vi "Main.vi"(11 "Module Admin":refnum<class "Delacor_lib_QMH_Module Admin.lvclass">) -> ()   [LabVIEW 2020, in "Logging.lvlib"]
doc: "This template is based off of the Queued Message Handler design pattern and the Queued Message Handler project template that ships with LabVIEW.\n\nThe main difference is that the queue is private to this module and communication between modules is performed via Broadcast and Request events.\n\nRequest events are wrapped in public API methods and are handled in the Event Handling Loop (EHL) of this VI. Any module can register for Broadcast events sent by this module. The EHL generates messages based on user interface actions.\n\nThe Message Handling Loop (MHL) processes messages generated by the EHL, or by other messages. The messages are string values, so new messages can be added easily to the Message Cases case structure in the MHL. Each message cluster can also provide an optional value for Message Data, which is a variant that can be converted to whatever message-specific data is required.\n_____\nBased on Delacor QMH Project Template 6.0.0.89."
uses:
  Logging.lvlib
  <vilib>/Delacor/Delacor QMH/Libraries/Module Admin_class/Delacor_lib_QMH_Module Admin.lvclass
  Module Data--cluster.ctl
  Stop Argument--cluster.ctl
  <vilib>/Delacor/Delacor QMH/Libraries/Message Queue_class/Delacor_lib_QMH_Message Queue.lvclass/Delacor_lib_QMH_Message Queue.ctl
  <vilib>/Delacor/Delacor QMH/Libraries/Module Admin_class/Delacor_lib_QMH_Module Admin.lvclass/Delacor_lib_QMH_Module Admin.ctl
  save tdms Argument--cluster.ctl
  <vilib>/Utility/miscctls.llb/LVPointTypeDef.ctl
  <vilib>/Delacor/Delacor QMH/Libraries/Message Queue_class/Delacor_lib_QMH_Enqueue Message (Single).vi
  <vilib>/Delacor/Delacor QMH/Libraries/Module Admin_class/Delacor_lib_QMH_Get External Launch.vi
  <vilib>/Utility/error.llb/Error Cluster From Error Code.vi
  <vilib>/ErrorRing/Error Ring.xnode
  <vilib>/Delacor/Delacor QMH/Libraries/Message Queue_class/Delacor_lib_QMH_Message Queue.lvclass
  Settings/Settings.lvlib
  Acquisition/Acquisition .lvlib
panel:
  out "data":waveform(dbl)[](array[waveform])
  in  "Save Button":bool
  out "error out":errorcluster
  out "Status":string
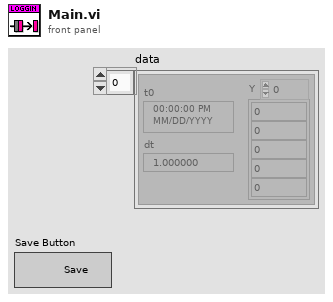
[diagram p1: front panel]
types:
  T1 = typedef "Logging.lvlib/Request Events--cluster.ctl" = cluster{"Stop Module":refnum<user-event>, "Show Panel":refnum<user-event>, "Hide Panel":refnum<user-event>, "Get Module Execution Status":refnum<user-event>, "Show Diagram":refnum<user-event>, "save tdms":refnum<user-event>}
  T2 = typedef "Acquisition .lvlib/Broadcast Events--cluster.ctl" = cluster{"Module Did Init":refnum<user-event>, "Status Updated":refnum<user-event>, "Error Reported":refnum<user-event>, "Module Did Stop":refnum<user-event>, "Update Module Execution Status":refnum<user-event>, "analog data":refnum<user-event>, "digital data":refnum<user-event>, "Digital Metdata has been acquired":refnum<user-event>}
  T3 = typedef "Settings.lvlib/Broadcast Events--cluster.ctl" = cluster{"Module Did Init":refnum<user-event>, "Status Updated":refnum<user-event>, "Error Reported":refnum<user-event>, "Module Did Stop":refnum<user-event>, "Update Module Execution Status":refnum<user-event>, "Config has been set":refnum<user-event>, "Prueba has been set":refnum<user-event>, "Digital has been set":refnum<user-event>}
  T4 = typedef "Logging.lvlib/Module Data--cluster.ctl" = cluster{"Status":string, "Nombre de la Prueba":string, "data":waveform(dbl)[], "data 2":u8[]}
  T5 = enum32{"invalid lock state", "Not Locked", "Locked (No Password)", "Password-protected"}
  T6 = typedef "Logging.lvlib/Stop Argument--cluster.ctl" = cluster{"Origin":string, "Exit via Stop Module Req?":bool, "Wait for Module to stop?":bool}
  T7 = typedef "Logging.lvlib/save tdms Argument--cluster.ctl" = cluster{"Boolean":bool}
  T8 = typedef "LVPointTypeDef.ctl" = cluster{"Horizontal":i16, "Vertical":i16}
  T9 = enum32{"Invalid", "Standard", "Closed", "Hidden", "Minimized", "Maximized"}
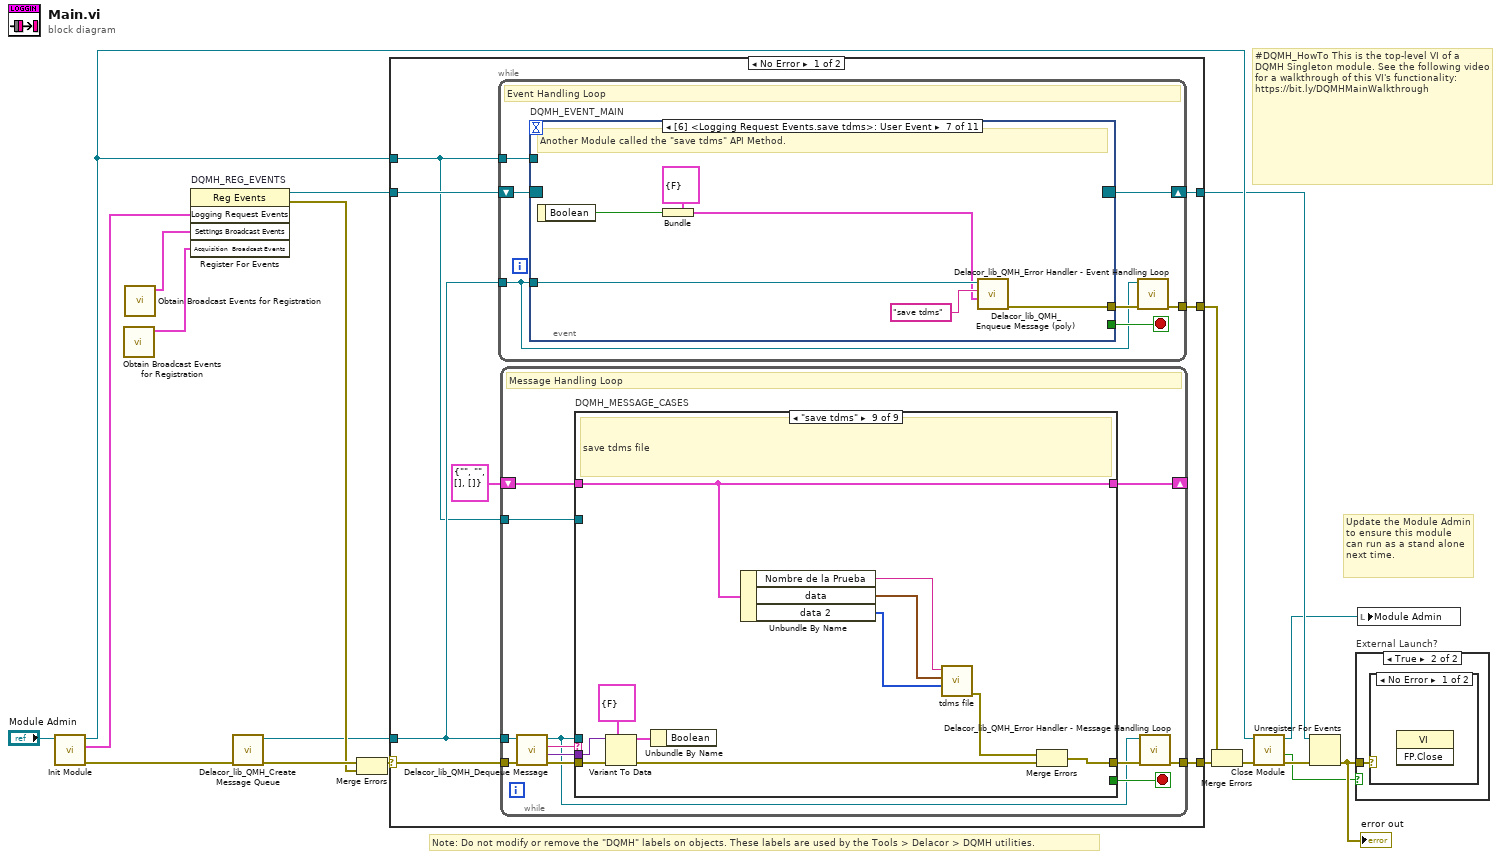
[diagram p0: block diagram]
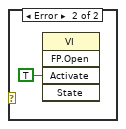
[diagram p3: hidden frame]
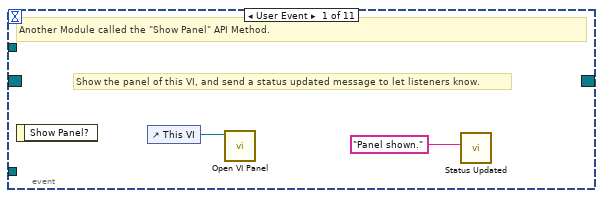
[diagram p4: hidden frame]
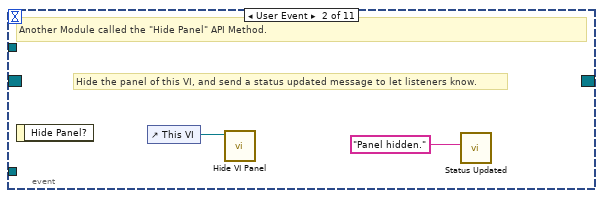
[diagram p5: hidden frame]
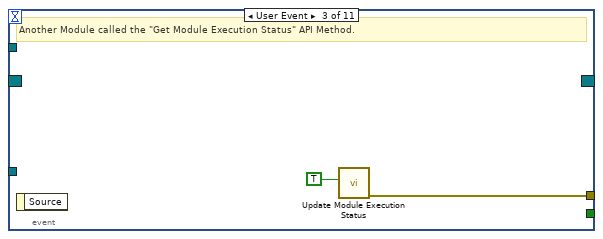
[diagram p6: hidden frame]
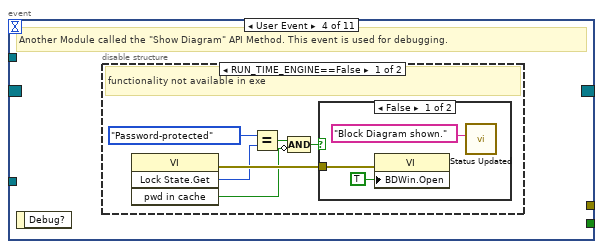
[diagram p7: hidden frame]
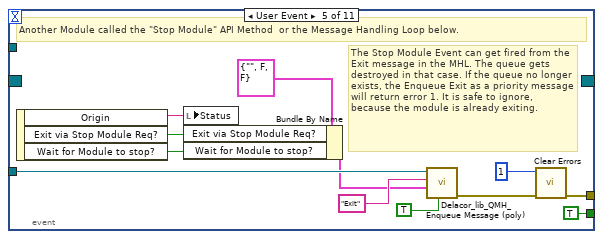
[diagram p10: hidden frame]
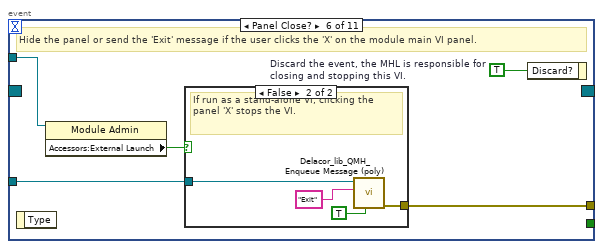
[diagram p11: hidden frame]
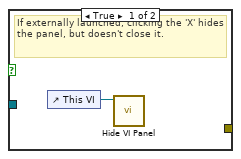
[diagram p12: hidden frame]
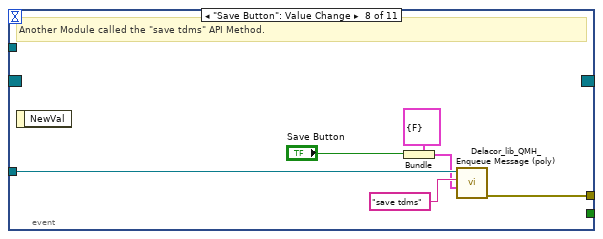
[diagram p13: hidden frame]
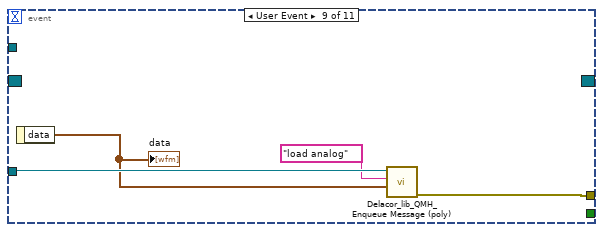
[diagram p14: hidden frame]
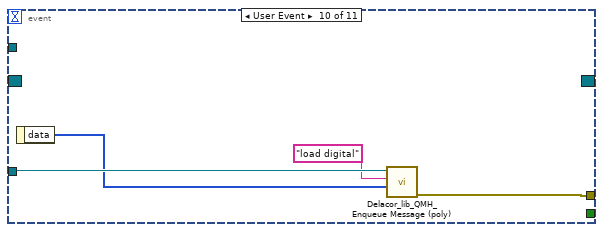
[diagram p15: hidden frame]
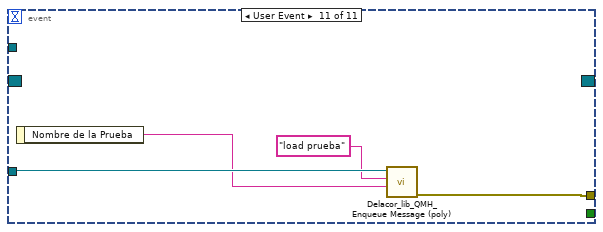
[diagram p16: hidden frame]
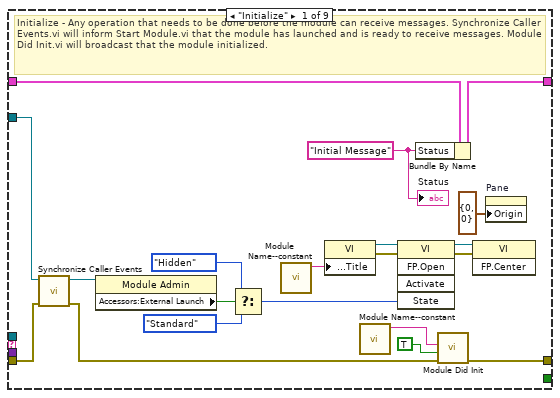
[diagram p17: hidden frame]
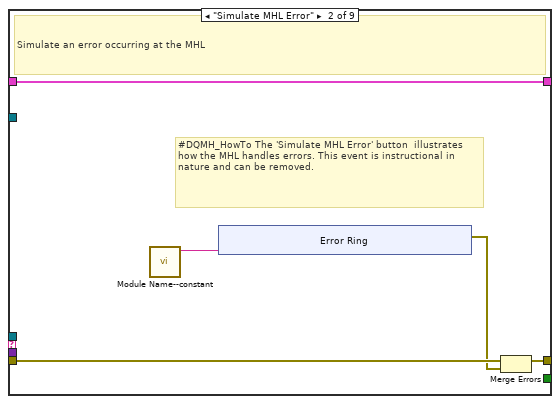
[diagram p18: hidden frame]
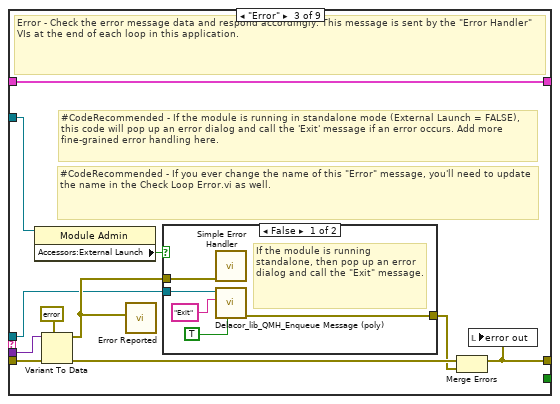
[diagram p19: hidden frame]
diagram:
  # "#DQMH_HowTo This is the top-level VI of a DQMH Singleton module. See the following video for a walkthrough of this VI's functionality: https://bit.ly/DQMHMainWalkthrough"
  # "Note: Do not modify or remove the \"DQMH\" labels on objects. These labels are used by the Tools > Delacor > DQMH utilities."
  # "Update the Module Admin to ensure this module can run as a stand alone next time."
  n1 = call "Init Module.vi"("Singleton Module Admin in"="Module Admin") -> ("error out"=w18:errorcluster, "Logging Request Events"=w7:T1, "Singleton Module Admin out"=w10:refnum<class "Delacor_lib_QMH_Module Admin.lvclass">)  [unwired: 8 in]
  n2 = call "Obtain Broadcast Events for Registration.vi"() -> ("Acquisition  Broadcast Events"=w1:T2)  [unwired: 9 in, 2 out]
  n3 = call "Obtain Broadcast Events for Registration.vi"() -> ("Settings Broadcast Events"=w2:T3)  [unwired: 9 in, 2 out]
  n4 = register-events "DQMH_REG_EVENTS"(w7, w2, w1) -> (reference out=w8:refnum<event-registration>, error out=w11:errorcluster)  [unwired: 2 in]
  n5 = call <vilib>:"Delacor_lib_QMH_Create Message Queue.vi"("error in"=w18) -> ("error out"=w13:errorcluster, "Message Queue"=w6:refnum<class "Delacor_lib_QMH_Message Queue.lvclass">)  [unwired: 9 in]
  n6 = Merge Errors(w13, w11) -> (w12:errorcluster)
  n7 = case shown="No Error" w12 {
    selector: w12 -> [w25 w225]
    tunnel: [w27 w224] -> w19
    tunnel: [w24 w230] -> w9
    tunnel: w8 -> [w22 w230]
    tunnel: w6 -> [w21 w223]
    tunnel: [w26 _] -> w16
    tunnel: w10 -> [w20 w226]
    frame No Error {
      n8 = while {
        tunnel: w21 -> [w28]
        shift-right: [w31] -> w24
        shift-left: w22 -> [w32]
        tunnel: [w33] -> w26
        tunnel: w20 -> [w29]
        stop <- w30 stop-if-true
        # "Event Handling Loop"
        n9 = event "DQMH_EVENT_MAIN" shown="[6] <Logging Request Events.save tdms>: User Event" {
          selector: w32 -> [_ _ _ _ _ _ _ _ _ _ _]
          dyn-events: [_ _ _ _ _ _ _ _ _ _ _] -> w31
          timeout: _ -> [_ _ _ _ _ _ _ _ _ _ _]
          tunnel: [_ _ _ _ TRUE ("Discard?") _ _ _ _ _ _] -> w30
          tunnel: w28 -> [_ _ _ _ w57 w64 w77 w83 w86 w90 w94]
          tunnel: [_ _ w40 _ w60 w66 w72 w79 w87 w91 w95] -> w34
          tunnel: w29 -> [_ _ _ _ _ w63 _ _ _ _ _]
          event User Event {
            # "Show the panel of this VI, and send a status updated message to let listeners know."
            # "Another Module called the \"Show Panel\" API Method."
            n10 = event-data() -> ()  [unwired: 1 in, 1 out]
            n11 = control-ref of="This VI"() -> (w36:refnum<vi>)
            n12 = call "Open VI Panel.vi"("VI"=w36) -> ()  [unwired: 10 in, 1 out]
            n13 = call "Status Updated.vi"("Status"="Panel shown." ("format string")) -> ()  [unwired: 10 in, 1 out]
          }
          event User Event {
            # "Hide the panel of this VI, and send a status updated message to let listeners know."
            # "Another Module called the \"Hide Panel\" API Method."
            n14 = event-data() -> ()  [unwired: 1 in, 1 out]
            n15 = control-ref of="This VI"() -> (w38:refnum<vi>)
            n16 = call "Hide VI Panel.vi"("VI"=w38) -> ()  [unwired: 10 in, 1 out]
            n17 = call "Status Updated.vi"("Status"="Panel hidden." ("format string")) -> ()  [unwired: 10 in, 1 out]
          }
          event User Event {
            # "Another Module called the \"Get Module Execution Status\" API Method."
            n18 = event-data() -> ()  [unwired: 1 in, 1 out]
            n19 = call "Update Module Execution Status.vi"("Running?"=TRUE) -> ("error out"=w40:errorcluster)  [unwired: 10 in]
          }
          event User Event {
            # "Another Module called the \"Show Diagram\" API Method. This event is used for debugging."
            n20 = event-data() -> ()  [unwired: 1 in, 1 out]
            n21 = disable-structure shown="RUN_TIME_ENGINE==False" {
              frame condition #0 (active) {
                # "functionality not available in exe"
                n22 = invoke class="VI" method="Lock State.Get"() -> (error out=w46:errorcluster, "Get Lock State"=w45:T5, "pwd in cache"=w42:bool)  [unwired: 4 in, 1 out]
                n23 = Equal?(x=T5."Password-protected", y=w45) -> (x = y?=w43:bool)
                n24 = Compound Arithmetic op=AND(w43, invert w42) -> (w41:bool)
                n25 = case shown="False" w41 {
                  tunnel: w46 -> [w49 _]
                  frame False {
                    n26 = property class="VI"(error in=w49, "BDWin.Open"=TRUE ("Block Diagram Window:Open")) -> ()  [unwired: 1 in, 2 out]
                    n27 = call "Status Updated.vi"("Status"="Block Diagram shown." ("format string")) -> ()  [unwired: 10 in, 1 out]
                  }
                  frame True {
                    # "Password-protected VI, and the password is not in the cache. Do not show the diagram."
                  }
                }
              }
              frame condition #1 {
              }
            }
          }
          event User Event {
            # "The Stop Module Event can get fired from the Exit message in the MHL. The queue gets destroyed in that case. If the queue no longer exists, the Enqueue Exit as a priority message will return error 1. It is safe to ignore, because the module is already exiting."
            # "Another Module called the \"Stop Module\" API Method  or the Message Handling Loop below."
            n28 = event-data() -> ("Origin"=w56:string, "Exit via Stop Module Req?"=w52:bool, "Wait for Module to stop?"=w51:bool)  [unwired: 1 in]
            n29 = local write "Status"(w56) -> ()
            n30 = Bundle By Name(cluster=T6 {"Origin"="", "Exit via Stop Module Req?"=FALSE, "Wait for Module to stop?"=FALSE} ("Stop Argument"), "Exit via Stop Module Req?"=w52, "Wait for Module to stop?"=w51) -> (w50:T6)
            n31 = call-poly <vilib>:"Delacor_lib_QMH_Enqueue Message (poly).vi"("Priority Message? (F)"=TRUE, "Message Data"=w50, "Message"="Exit", "Message Queue in"=w57) -> ("error out"=w61:errorcluster)  [unwired: 6 in, 1 out]
            n32 = call <vilib>:"Clear Errors.vi"("error in (no error)"=w61, "specific error code to clear (0: all)"=1) -> ("error out"=w60:errorcluster)  [unwired: 4 in, 1 out]
          }
          event Panel Close? {
            w65 = TRUE  # Discard the event, the MHL is responsible for closing and stopping this VI.
            # "Hide the panel or send the 'Exit' message if the user clicks the 'X' on the module main VI panel."
            n33 = event-data() -> ()  [unwired: 1 in, 1 out]
            n34 = property class="Module Admin"(reference=w63) -> ("Accessors:External Launch"=w62:bool)  [unwired: 1 in, 2 out]
            n35 = case shown="False" w62 {
              tunnel: w64 -> [_ w70]
              tunnel: [_ w71] -> w66
              frame True {
                # "If externally launched, clicking the 'X' hides the panel, but doesn't close it."
                n36 = control-ref of="This VI"() -> (w67:refnum<vi>)
                n37 = call "Hide VI Panel.vi"("VI"=w67) -> ()  [unwired: 10 in, 1 out]
              }
              frame False {
                # "If run as a stand-alone VI, clicking the panel 'X' stops the VI."
                n38 = call-poly <vilib>:"Delacor_lib_QMH_Enqueue Message (poly).vi"("Priority Message? (F)"=TRUE, "Message"="Exit", "Message Queue in"=w70) -> ("error out"=w71:errorcluster)  [unwired: 7 in, 1 out]
              }
            }
            n39 = event-data("Discard?"=w65) -> ()  [unwired: 1 in, 1 out]
          }
          event User Event {
            # "Another Module called the \"save tdms\" API Method."
            n40 = event-data() -> ("Boolean"=w73:bool)  [unwired: 1 in]
            n41 = Bundle(cluster=T7 {"Boolean"=FALSE} ("save tdms Argument"), "Boolean"=w73) -> (w74:T7)
            n42 = call-poly <vilib>:"Delacor_lib_QMH_Enqueue Message (poly).vi"("Message Data"=w74, "Message"="save tdms", "Message Queue in"=w77) -> ("error out"=w72:errorcluster)  [unwired: 7 in, 1 out]
          }
          event "Save Button": Value Change {
            # "Another Module called the \"save tdms\" API Method."
            n43 = event-data() -> ()  [unwired: 1 in, 1 out]
            n44 = Bundle(cluster=T7 {"Boolean"=FALSE} ("save tdms Argument"), "Boolean"="Save Button") -> (w80:T7)
            n45 = call-poly <vilib>:"Delacor_lib_QMH_Enqueue Message (poly).vi"("Message Data"=w80, "Message"="save tdms", "Message Queue in"=w83) -> ("error out"=w79:errorcluster)  [unwired: 7 in, 1 out]
          }
          event User Event {
            n46 = event-data() -> ("data"=w84:waveform(dbl)[])  [unwired: 1 in]
            "data" <- w84
            n47 = call-poly <vilib>:"Delacor_lib_QMH_Enqueue Message (poly).vi"("Message Data"=w84, "Message"="load analog", "Message Queue in"=w86) -> ("error out"=w87:errorcluster)  [unwired: 7 in, 1 out]
          }
          event User Event {
            n48 = event-data() -> ("data"=w88:u8[])  [unwired: 1 in]
            n49 = call-poly <vilib>:"Delacor_lib_QMH_Enqueue Message (poly).vi"("Message Data"=w88, "Message"="load digital", "Message Queue in"=w90) -> ("error out"=w91:errorcluster)  [unwired: 7 in, 1 out]
          }
          event User Event {
            n50 = event-data() -> ("Nombre de la Prueba"=w93:string)  [unwired: 1 in]
            n51 = call-poly <vilib>:"Delacor_lib_QMH_Enqueue Message (poly).vi"("Message Data"=w93, "Message"="load prueba", "Message Queue in"=w94) -> ("error out"=w95:errorcluster)  [unwired: 7 in, 1 out]
          }
        }
        n52 = call-dynamic "Delacor_lib_QMH_Error Handler - Event Handling Loop.vi"("error in"=w34, "Message Queue in"=w28) -> ("dup error in"=w33:errorcluster)  [unwired: 8 in, 1 out]
      }
      n53 = while {
        tunnel: w21 -> [w98]
        shift-right: [w102] -> _
        shift-left: T4 {"Status"="", "Nombre de la Prueba"="", "data"=[], "data 2"=[]} ("Data Cluster") -> [w103]
        tunnel: w25 -> [w106]
        tunnel: [w104] -> w27
        tunnel: w20 -> [w96]
        stop <- w101 stop-if-true
        # "Message Handling Loop"
        n54 = call-dynamic "Delacor_lib_QMH_Dequeue Message.vi"("error in"=w106, "Message Queue in"=w98) -> ("error out"=w105:errorcluster, "Message Data"=w99:variant, "Message"=w100:string, "Message Queue out"=w97:refnum<class "Delacor_lib_QMH_Message Queue.lvclass">)  [unwired: 6 in]
        n55 = case "DQMH_MESSAGE_CASES" shown="\"save tdms\"" w100 {
          selector: w100 -> [_ _ _ _ w172 _ _ _ _]
          tunnel: w97 -> [_ _ w142 w164 _ w186 w195 _ _]
          tunnel: w105 -> [w125 w132 w149 w170 w174 w194 w204 w211 w222]
          tunnel: [w123 w131 w145 w167 w175 w188 w197 w210 w216] -> w107
          tunnel: w103 -> [w114 w129 w144 w163 w173 w191 w202 w208 w217]
          tunnel: [w113 w129 w144 w163 w173 w189 w201 w205 w217] -> w102
          tunnel: [_ _ _ w162 _ _ _ _ _] -> w101
          tunnel: w99 -> [_ _ w143 w161 _ w193 w203 w209 w220]
          tunnel: w96 -> [w115 _ w141 w156 _ _ _ _ _]
          frame "Initialize" {
            w109 = "Initial Message" ("Initial Message")
            # "Initialize - Any operation that needs to be done before the module can receive messages. Synchronize Caller Events.vi will inform Start Module.vi that the module has launched and is ready to receive messages. Module Did Init.vi will broadcast that the module initialized."
            n56 = call "Synchronize Caller Events.vi"("error in (no error)"=w125, "Singleton Module Admin in"=w115) -> ("error out"=w124:errorcluster, "Singleton Module Admin out"=w110:refnum<class "Delacor_lib_QMH_Module Admin.lvclass">)  [unwired: 8 in]
            n57 = property class="Module Admin"(reference=w110) -> ("Accessors:External Launch"=w119:bool)  [unwired: 1 in, 2 out]
            n58 = Select(t=T9."Hidden" ("State"), s=w119, f=T9."Standard" ("State")) -> (s? t:f=w116:T9)
            n59 = call "Module Name--constant.vi"() -> ("Module Name"=w122:string)  [unwired: 11 in]
            n60 = property class="VI"("Front Panel.Title"=w122) -> (reference out=w121:refnum<vi>, error out=w127:errorcluster)  [unwired: 2 in]
            n61 = call "Module Name--constant.vi"() -> ("Module Name"=w111:string)  [unwired: 11 in]
            n62 = invoke class="VI" method="FP.Open"(reference=w121, error in=w127, "State"=w116) -> (reference out=w120:refnum<vi>, error out=w126:errorcluster)  [unwired: 2 in, 3 out]
            n63 = Bundle By Name(cluster=w114, "Status"=w109) -> (w113:T4)
            n64 = call "Module Did Init.vi"("error in (no error)"=w124, "Initialized?"=TRUE, "Origin"=w111) -> ("error out"=w123:errorcluster)  [unwired: 8 in]
            n65 = invoke class="VI" method="FP.Center"(reference=w120, error in=w126) -> ()  [unwired: 1 in, 3 out]
            n66 = property on="Pane" class="Pane"("Origin"=T8 {"Horizontal"=0, "Vertical"=0}) -> ()  [unwired: 2 in, 2 out]
            "Status" <- w109
          }
          frame "Simulate MHL Error" {
            # "#DQMH_HowTo The 'Simulate MHL Error' button  illustrates how the MHL handles errors. This event is instructional in nature and can be removed."
            # "Simulate an error occurring at the MHL"
            n67 = call "Module Name--constant.vi"() -> ("Module Name"=w128:string)  [unwired: 11 in]
            n68 = xnode "Error Ring"("parameter 0"=w128) -> ("error out"=w130:errorcluster)
            n69 = Merge Errors(w132, w130) -> (w131:errorcluster)
          }
          frame "Error" {
            # "#CodeRecommended - If you ever change the name of this \"Error\" message, you'll need to update the name in the Check Loop Error.vi as well."
            # "#CodeRecommended - If the module is running in standalone mode (External Launch = FALSE), this code will pop up an error dialog and call the 'Exit' message if an error occurs. Add more fine-grained error handling here."
            # "Error - Check the error message data and respond accordingly. This message is sent by the \"Error Handler\" VIs at the end of each loop in this application."
            n70 = property class="Module Admin"(reference=w141) -> ("Accessors:External Launch"=w140:bool)  [unwired: 1 in, 2 out]
            n71 = Variant To Data(error in=w149, type=errorcluster {"status"=FALSE, "code"=0, "source"=""} ("error constant"), Variant=w143) -> (data=w150:errorcluster, error out=w147:errorcluster)
            n72 = call "Error Reported.vi"("Error"=w150) -> ()  [unwired: 10 in, 1 out]
            n73 = case shown="False" w140 {
              tunnel: [w155 _] -> w146
              tunnel: w142 -> [w153 _]
              tunnel: w150 -> [w154 _]
              frame False {
                # "If the module is running standalone, then pop up an error dialog and call the \"Exit\" message."
                n74 = call <vilib>:"Simple Error Handler.vi"("error in (no error)"=w154) -> ()  [unwired: 4 in, 5 out]
                n75 = call-poly <vilib>:"Delacor_lib_QMH_Enqueue Message (poly).vi"("Priority Message? (F)"=TRUE, "Message"="Exit", "Message Queue in"=w153) -> ("error out"=w155:errorcluster)  [unwired: 7 in, 1 out]
              }
              frame True {
                # "If the module was launched externally, calling the Error Reported broadcast VI is the only action performed by the \"Error\" message. The module's caller can then process the error appropriately."
              }
            }
            n76 = Merge Errors(w147, w146) -> (w145:errorcluster)
            n77 = local write "error out"(w145) -> ()
          }
          frame "Exit" {
            w160 = 91  # 91: not all Exit messages will have an argument
            w162 = TRUE  # Stop the VI
            # "Release the message queue reference"
            # "#CodeNeeded - Add any required cleanup code here"
            # "Exit - Exit the application."
            n78 = Variant To Data(error in=w170, type=T6 {"Origin"="", "Exit via Stop Module Req?"=FALSE, "Wait for Module to stop?"=FALSE} ("Stop Argument"), Variant=w161) -> (data=w158:T6, error out=w166:errorcluster)
            n79 = call <vilib>:"Clear Errors.vi"("error in (no error)"=w166, "specific error code to clear (0: all)"=w160) -> ("error out"=w169:errorcluster)  [unwired: 4 in, 1 out]
            n80 = control-ref of="This VI"() -> (w157:refnum<vi>)
            n81 = call-dynamic "Delacor_lib_QMH_Release Message Queue.vi"("error in"=w169, "Message Queue"=w164) -> ("error out"=w168:errorcluster)  [unwired: 9 in]
            n82 = call "Handle Exit.vi"("Stop Argument"=w158, "Admin in"=w156, "VI reference"=w157) -> ("error out"=w165:errorcluster)  [unwired: 7 in, 1 out]
            n83 = Merge Errors(w168, w165) -> (w167:errorcluster)
            n84 = call "Stop Module.vi"() -> ()  [unwired: 11 in, 1 out]
          }
          frame Default {
            # "'Default' case only runs if there is a message that isn't defined in any of the other cases.  Output a programming error."
            n85 = call "Module Name--constant.vi"() -> ("Module Name"=w171:string)  [unwired: 11 in]
            n86 = xnode "Error Ring"("parameter 0"=w172, "parameter 1"=w171) -> ("error out"=w176:errorcluster)
            n87 = Merge Errors(w174, w176) -> (w175:errorcluster)
          }
          frame "load analog" {
            n88 = Variant To Data(error in=w194, type=waveform(dbl)[] [] ("data"), Variant=w193) -> (data=w190:waveform(dbl)[], error out=w187:errorcluster)
            n89 = Bundle By Name(cluster=w191, "data"=w190) -> (w189:T4)
            n90 = call-poly <vilib>:"Delacor_lib_QMH_Enqueue Message (poly).vi"("error in"=w187, "Message"="save tdms", "Message Queue in"=w186) -> ("error out"=w188:errorcluster)  [unwired: 7 in, 1 out]
          }
          frame "load digital" {
            n91 = Variant To Data(error in=w204, type=u8[] [] ("data"), Variant=w203) -> (data=w199:u8[], error out=w196:errorcluster)
            n92 = Bundle By Name(cluster=w202, "data 2"=w199) -> (w201:T4)
            n93 = call-poly <vilib>:"Delacor_lib_QMH_Enqueue Message (poly).vi"("error in"=w196, "Message"="save tdms", "Message Queue in"=w195) -> ("error out"=w197:errorcluster)  [unwired: 7 in, 1 out]
          }
          frame "load prueba" {
            n94 = Variant To Data(error in=w211, type="" ("Nombre de la Prueba"), Variant=w209) -> (data=w207:string, error out=w210:errorcluster)
            n95 = Bundle By Name(cluster=w208, "Nombre de la Prueba"=w207) -> (w205:T4)
          }
          frame "save tdms" {
            # "save tdms file"
            n96 = Variant To Data(error in=w222, type=T7 {"Boolean"=FALSE} ("save tdms Argument"), Variant=w220) -> (data=w218:T7, error out=w221:errorcluster)
            n97 = Unbundle By Name(w218) -> ()  [unwired: 1 out]
            n98 = Unbundle By Name(w217) -> ("Nombre de la Prueba"=w214:string, "data"=w213:waveform(dbl)[], "data 2"=w212:u8[])
            n99 = call "tdms file.vi"("data 2"=w212, "analog data"=w213, "String"=w214) -> ("error out"=w215:errorcluster)  [unwired: 8 in]
            n100 = Merge Errors(w215, w221) -> (w216:errorcluster)
          }
        }
        n101 = call-dynamic "Delacor_lib_QMH_Error Handler - Message Handling Loop.vi"("error in"=w107, "Message Queue in"=w97) -> ("dup error in"=w104:errorcluster)  [unwired: 8 in, 1 out]
      }
    }
    frame Error {
      # "Synchronize Caller Events.vi will inform Start Module.vi that the module has launched and will let the code calling Start Module.vi register for broadcasts and would permit the caller receive the broadcast that an error occurred at launch time."
      n102 = call-dynamic "Delacor_lib_QMH_Release Message Queue.vi"("error in"=w225, "Message Queue"=w223) -> ("error out"=w224:errorcluster)  [unwired: 9 in]
      n103 = call "Synchronize Caller Events.vi"("Singleton Module Admin in"=w226) -> ("error out"=w231:errorcluster)  [unwired: 9 in, 1 out]
      n104 = call "Module Name--constant.vi"() -> ("Module Name"=w229:string)  [unwired: 11 in]
      n105 = Format Into String(format string="An error occurred during initialization. %s is no longer running.", w229) -> (resulting string=w227:string)  [unwired: 2 in, 1 out]
      n106 = Merge Errors(w224, w231) -> (w232:errorcluster)
      n107 = call "Error Reported.vi"("Additional Information"=w227, "Error"=w232) -> ()  [unwired: 9 in, 1 out]
      n108 = call "Stop Module.vi"() -> ()  [unwired: 11 in, 1 out]
      n109 = call "Stop Module.vi"() -> ()  [unwired: 11 in, 1 out]
    }
  }
  n110 = Merge Errors(w16, w19) -> (w15:errorcluster)
  n111 = call "Close Module.vi"("error in (no error)"=w15, "Module Admin in"=w10) -> ("error out"=w17:errorcluster, "External Launch"=w3:bool, "Module Admin out"=w4:refnum<class "Delacor_lib_QMH_Module Admin.lvclass">)  [unwired: 7 in]
  n112 = Unregister For Events(event registration refnum=w9, error in=w17) -> (error out=w14:errorcluster)
  "error out" <- w14
  n113 = case "External Launch?" shown="True" w3 {
    tunnel: w14 -> [_ w233]
    frame False {
    }
    frame True {
      n114 = case shown="No Error" w233 {
        frame No Error {
          n115 = invoke class="VI" method="FP.Close"() -> ()  [unwired: 3 in, 3 out]
        }
        frame Error {
          n116 = invoke class="VI" method="FP.Open"("Activate"=TRUE ("Activate?")) -> ()  [unwired: 4 in, 5 out]
        }
      }
    }
  }
  n117 = local write "Module Admin"(w4) -> ()
